vi "NXT_HINDBRAIN Servo Data To String.vi"(1 "_motorCommands":T1={"_rudderCommand"=7, "_propCommand"=7, "_irServoCommand"=7}) -> (0 "String":string)   [LabVIEW 2012, in "Tugboat.lvrbt"]
uses:
  Tugboat.lvrbt
  motorCommands_t.ctl
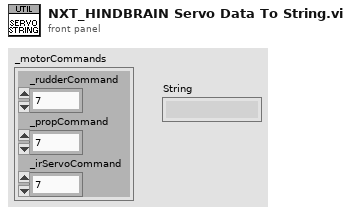
[diagram p1: front panel]
types:
  T1 = typedef "motorCommands_t.ctl" = cluster{"_rudderCommand":i8, "_propCommand":i8, "_irServoCommand":i8}
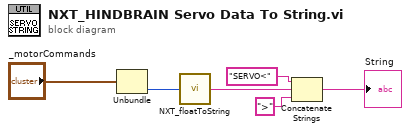
[diagram p0: block diagram]
diagram:
  n1 = Unbundle("_motorCommands") -> ("_irServoCommand"=w2:i8)  [unwired: 2 out]
  n2 = call <vilib>:"NXT_floatToString.vi"("number"=w2) -> ("string"=w4:string)
  n3 = Concatenate Strings("SERVO<" ("string"), w4, ">" ("string")) -> (→"String":string)
